vi "User Interface.vi"(10 "Test File Path":path=path "") -> ()   [LabVIEW 2020, in "Execution UI V2.lvclass"]
uses:
  Execution UI V2.lvclass
  <vilib>/Utility/miscctls.llb/LVNodeAndColumnTypeDef.ctl
  Application Framework/Process Classes/Process/Process.lvclass/Process.ctl
  Private/TypeDefs/Execution State.ctl
  Execution UI V2.lvclass/Execution UI V2.ctl
  Framework/Result Types/Case Result/Test Case Result.ctl
  Framework/Result Types/Method Result/Method Result.ctl
  Result/Status.ctl
  Framework/Result Types/Assertion Result/Assertion Result.ctl
  Framework/Result Types/Assertion Result/Public/TypeDefs/Assertion Type.ctl
  Framework/Result Types/Suite Results/Test Suite Result.ctl
  Result Model/Tree Item Filter.ctl
  Test Tree/Test Tree.lvclass
  Application Framework/Process Classes/Process/Public/Accessors/Read Process Name.vi
  C:/Git/astemes-lunit/source/Application Framework/Process Classes/Process/Process.lvclass
  <vilib>/Utility/error.llb/Error Cluster From Error Code.vi
  Framework/Result View/Result View.vi
  Application Framework/Process Classes/Error Handler/Private/SubVIs/Get Error Queue Name.vi
  <vilib>/Platform/browser.llb/Open URL in Default Browser (string).vi
  Framework/Result Types/Case Result/Test Case Result.lvlib
  Framework/Result Types/Method Result/Method Result.lvlib
  Framework/Result Types/Suite Results/Test Suite Result.lvlib
  Application Framework/Process Classes/Process/Process.lvclass
  Application Framework/Process Classes/Error Handler/Error Handler.lvclass
  Framework/Test Result View/Test Result View.lvclass
  Framework/Result Types/Assertion Result/Assertion Result.lvlib
  Result/Result.lvlib
  Result Table/Result Table V2.lvclass
  Result Model/Result Model.lvclass
panel:
  in  "Refresh":bool
  in  "Run Single Test":bool
  in  "Stop":bool
  in  "Run All Tests":bool
  in  "Eject":bool
  in  "Save":bool
  in  "Collapse":bool
  in  "Expand":bool
  out "Progress bar":dbl(slide) scale=0.0..100.0
  out "Results":i32(listbox)=-1
  in  "Test Results":string[](tree)
  in  "Filter fails":bool
  out "Description":string
  out "Status":string
  out "error out":errorcluster
  in  "error in (no error)":errorcluster
  # "1"
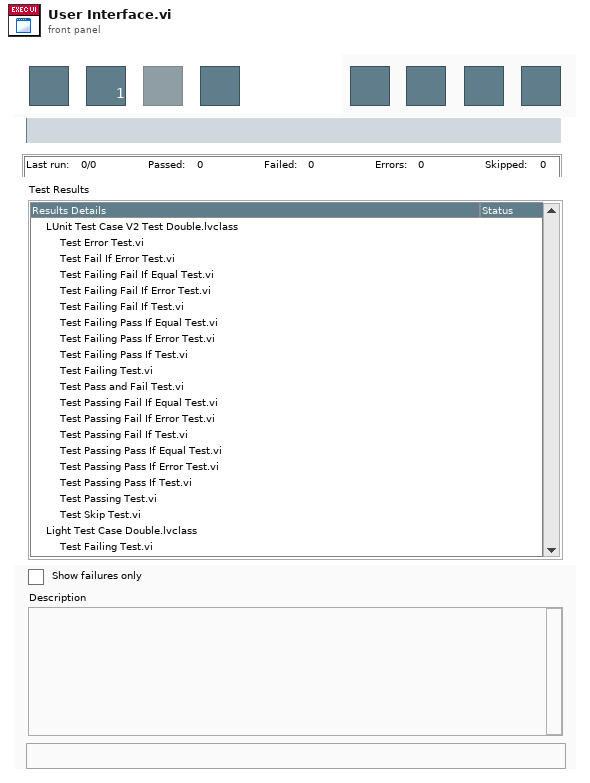
[diagram p1: front panel]
types:
  T1 = typedef "Execution UI V2.lvclass/Execution State.ctl" = enum16{"Idle", "Running"}
  T2 = typedef "Test Case Result.lvlib/Test Case Result.ctl" = map{string, T3}
  T3 = typedef "Method Result.lvlib/Method Result.ctl" = cluster{"Test Case":string, "Test Method Name":string, "Status":T4, "Assertion Results":T5[], "Execution time":dbl, "Result String":string}
  T4 = typedef "Result.lvlib/Status.ctl" = enum16{"", "Passed", "Failed", "Error", "Skipped", "Setup Error", "Broken", "Teardown Error"}
  T5 = typedef "Assertion Result.lvlib/Assertion Result.ctl" = cluster{"Status":T4, "Message":string, "Description":string, "Assertion Type":T6}
  T6 = typedef "Result.lvlib/Assertion Type.ctl" = enum16{"None", "Pass", "Fail", "Skip", "Pass if Equal", "Fail if Equal", "Pass if Error", "Fail if Error", "Pass if", "Fail if"}
  T7 = typedef "Test Suite Result.lvlib/Test Suite Result.ctl" = cluster{"Test Suite ID":string, "Name":string, "Hostname":string, "Status":T4, "Execution time":dbl, "Start Time":timestamp, "Case Results":T2[]}
  T8 = typedef "Result Model.lvclass/Tree Item Filter.ctl" = enum16{"All", "Only Fails"}
  T9 = typedef "LVNodeAndColumnTypeDef.ctl" = cluster{"Node":string, "Column":i32}
  T10 = enum8{"Enabled", "Disabled", "Disabled and Grayed Out"}
  T11 = typedef "Assertion Result.lvlib/Status.ctl" = enum16{"Pass", "Fail", "Error", "Skipped", "Setup Error", "Broken", "Teardown Error"}
  T12 = enum32{"Invalid", "Standard", "Closed", "Hidden", "Minimized", "Maximized"}
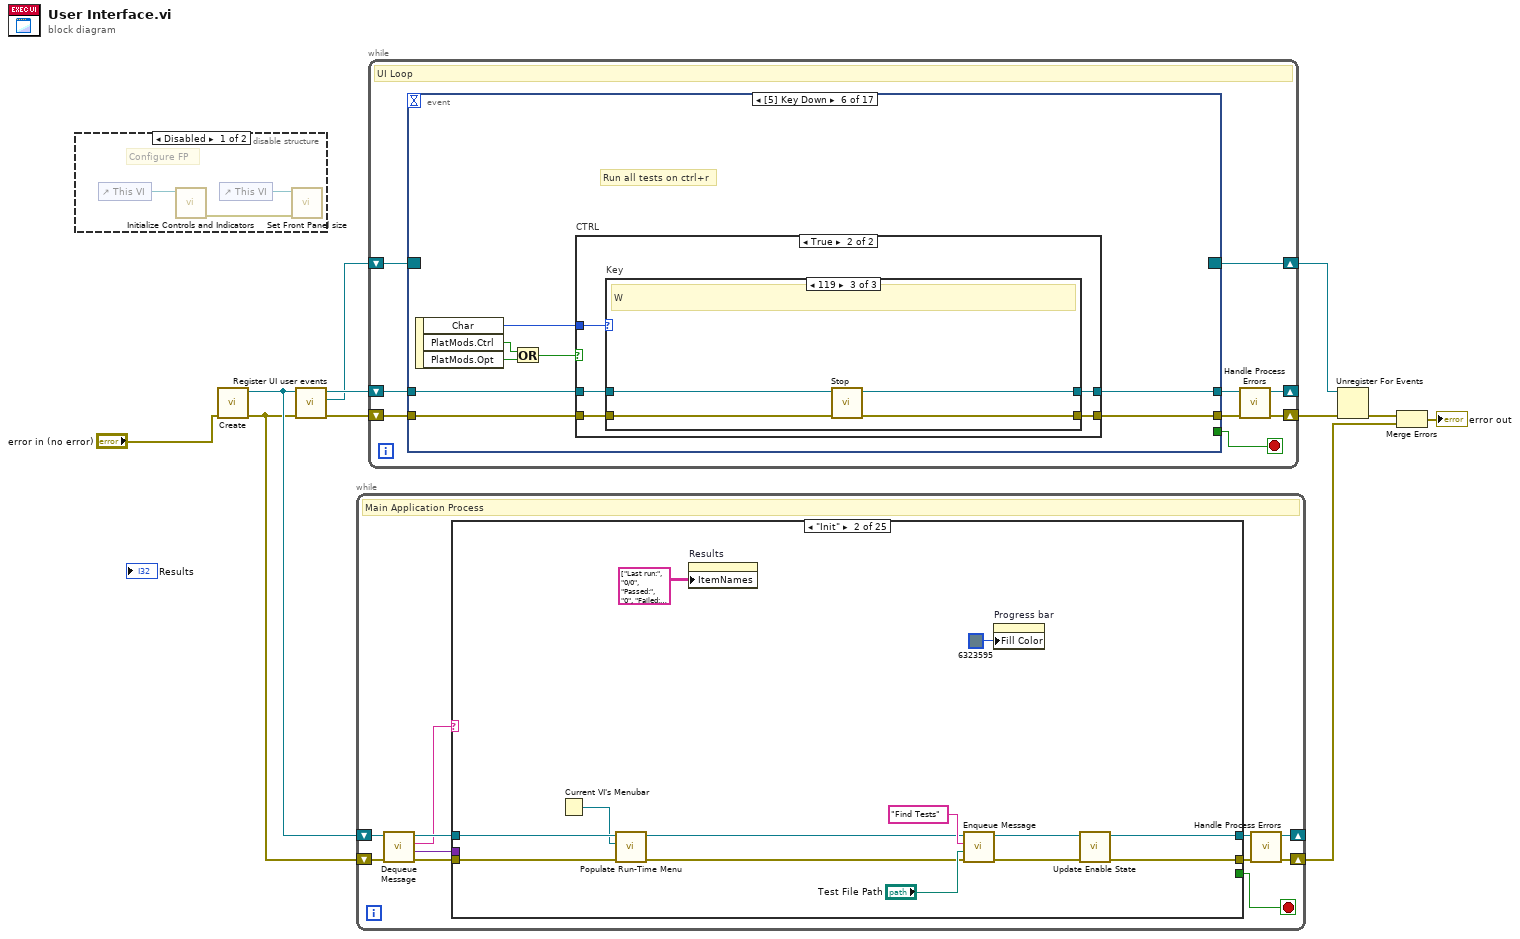
[diagram p0: block diagram]
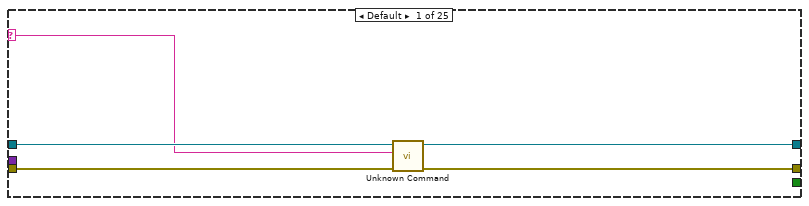
[diagram p2: hidden frame]
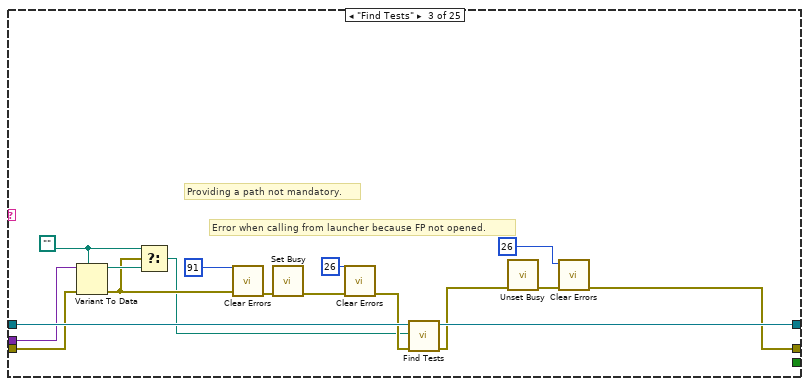
[diagram p3: hidden frame]
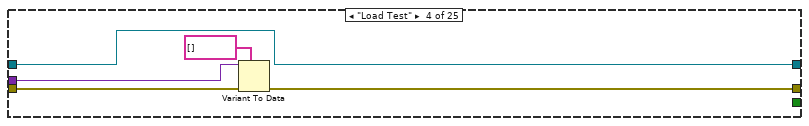
[diagram p4: hidden frame]
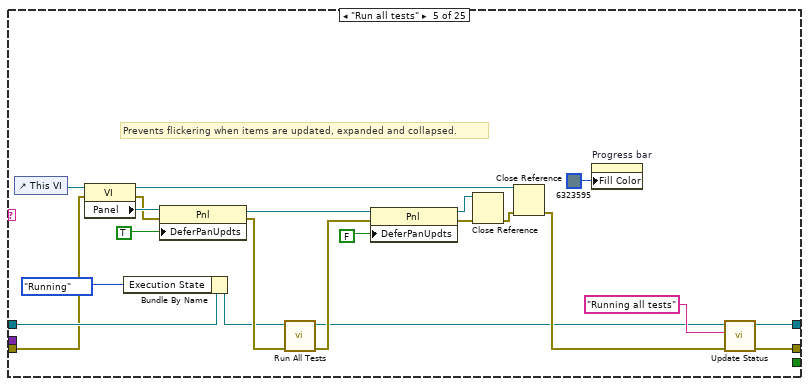
[diagram p5: hidden frame]
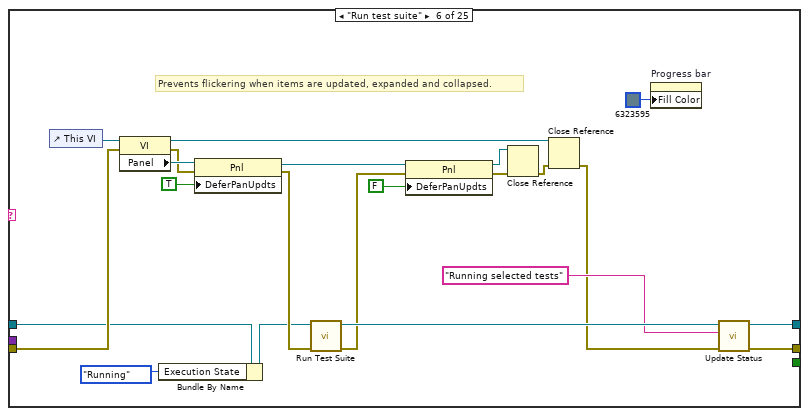
[diagram p6: hidden frame]
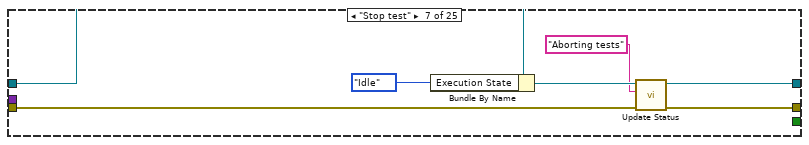
[diagram p7: hidden frame]
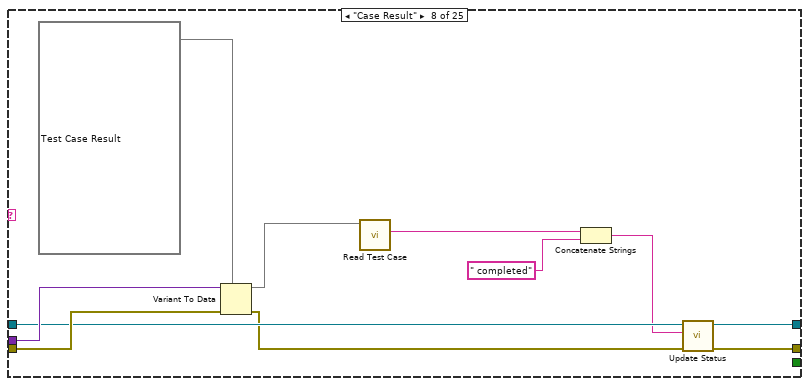
[diagram p8: hidden frame]
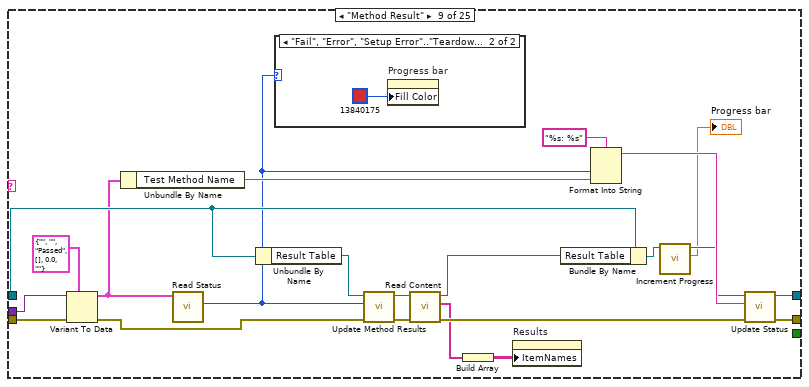
[diagram p9: hidden frame]
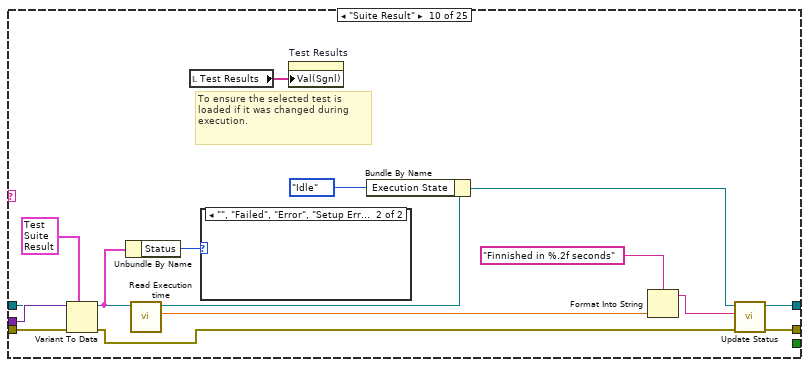
[diagram p11: hidden frame]
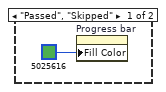
[diagram p12: hidden frame]
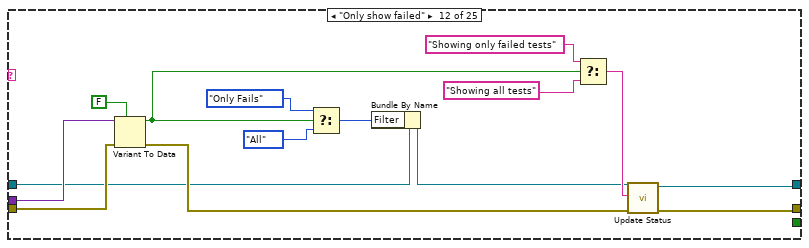
[diagram p14: hidden frame]
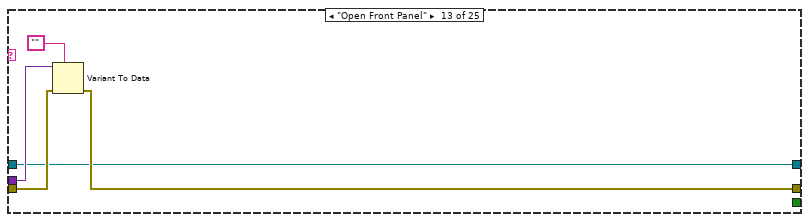
[diagram p15: hidden frame]
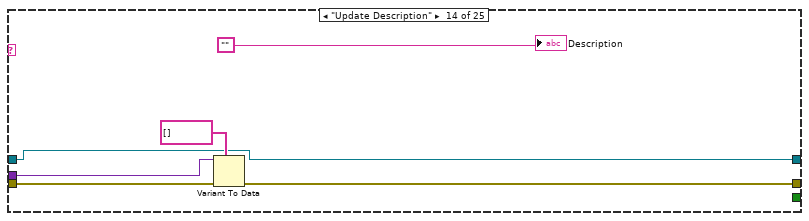
[diagram p16: hidden frame]
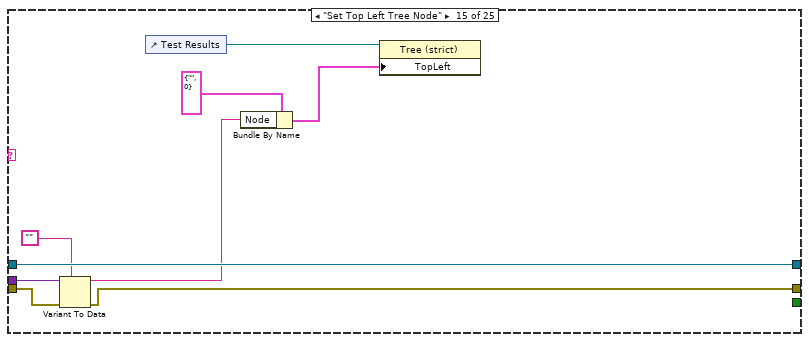
[diagram p17: hidden frame]
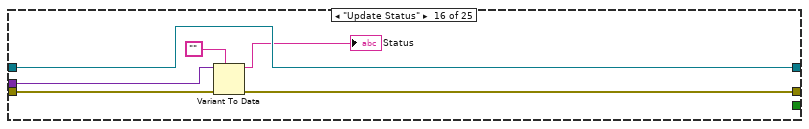
[diagram p18: hidden frame]
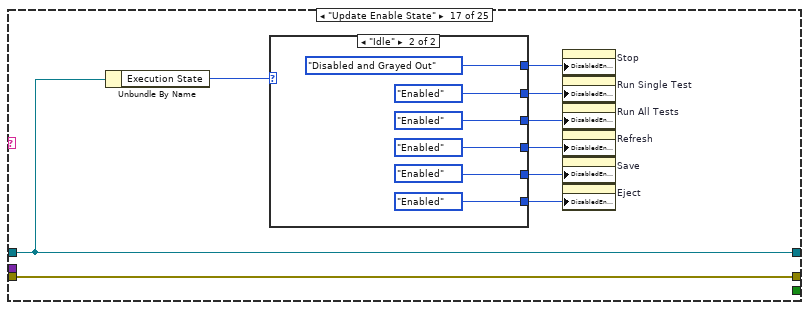
[diagram p19: hidden frame]
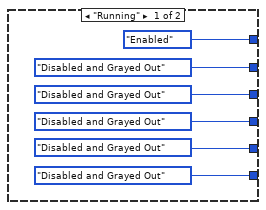
[diagram p20: hidden frame]
diagram:
  n1 = disable-structure shown="Disabled" {
    frame Disabled {
      # "Configure FP"
      n2 = control-ref of="This VI"() -> (w13:refnum<vi>)
      n3 = call "Initialize Controls and Indicators.vi"("VI in"=w13) -> ("error out"=w12:errorcluster)  [unwired: 10 in]
      n4 = control-ref of="This VI"() -> (w14:refnum<vi>)
      n5 = call "Set Front Panel size.vi"("error in (no error)"=w12, "VI in"=w14) -> ()  [unwired: 9 in, 1 out]
    }
    frame Enabled {
    }
  }
  n6 = call "Create.vi"("error in (no error)"="error in (no error)") -> ("error out"=w5:errorcluster, "Execution UI Out"=w6:refnum<class "Execution UI V2.lvclass">)  [unwired: 9 in]
  n7 = call "Register UI user events.vi"("error in (no error)"=w5, "Execution UI In"=w6) -> ("error out"=w10:errorcluster, "Event Registration Refnum"=w8:refnum<event-registration>, "Execution UI Out"=w11:refnum<class "Execution UI V2.lvclass">)  [unwired: 7 in]
  n8 = while {
    shift-right: [w16] -> w7
    shift-left: w5 -> [w24]
    shift-right: [w17] -> _
    shift-left: w6 -> [w25]
    stop <- w20 stop-if-true
    # "Main Application Process"
    n9 = call "Dequeue Message.vi"("error in (no error)"=w24, "Process In"=w25) -> ("error out"=w22:errorcluster, "Message Data"=w18:variant, "Message"=w19:string, "Process Out"=w23:refnum<class "Execution UI V2.lvclass">)  [unwired: 6 in]
    n10 = case shown="\"Init\"" w19 {
      selector: w19 -> [w26 _ _ _ _ _ _ _ _ _ _ _ _ _ _ _ _ _ w246 _ _ _ _ _ _]
      tunnel: w23 -> [w27 w35 w60 w65 w87 w89 w115 w124 w142 w158 w168 w174 w184 w190 w202 w206 w217 w244 w252 w259 w267 w275 w283 w289 w298]
      tunnel: [w28 w40 w57 w65 w86 w108 w110 w123 w146 w163 w168 w179 w184 w190 w202 w206 w217 w244 w252 w257 w265 w273 w281 w286 w302] -> w21
      tunnel: w22 -> [w29 w36 w53 w61 w79 w90 w114 w127 w149 w165 w167 w183 w188 w194 w203 w209 w218 w242 w251 w253 w264 w272 w280 w290 w292]
      tunnel: [w30 w39 w45 w62 w85 w107 w113 w122 w145 w162 w167 w178 w185 w191 w199 w205 w218 w243 w250 w258 w266 w274 w282 w285 w301] -> w15
      tunnel: [_ _ _ _ _ _ _ _ _ _ _ _ _ _ _ _ _ _ _ _ _ _ _ _ TRUE] -> w20
      tunnel: w18 -> [_ _ w56 w64 _ _ _ w126 w148 w164 _ w182 w187 w193 w201 w208 _ _ w249 _ _ _ _ _ _]
      frame Default {
        n11 = call "Unknown Command.vi"("error in (no error)"=w29, "String"=w26, "Process In"=w27) -> ("error out"=w30:errorcluster, "Process Out"=w28:refnum<class "Execution UI V2.lvclass">)  [unwired: 7 in]
      }
      frame "Init" {
        n12 = Current VI's Menubar() -> (w32:refnum<k9>)
        n13 = call "Populate Run-Time Menu.vi"("error in (no error)"=w36, "Menu in"=w32, "Execution UI"=w35) -> ("error out"=w34:errorcluster, "Execution UI"=w33:refnum<class "Execution UI V2.lvclass">)  [unwired: 7 in]
        n14 = property on="Results" class="MCListbox (strict)"("ItemNames"=string[][] [["Last run:", "0/0", "Passed:", "0", "Failed:", "0", "Errors:", "0", "Skipped:", "0"]] ("Result Texts")) -> ()  [unwired: 2 in, 2 out]
        n15 = call "Enqueue Message.vi"("error in (no error)"=w34, "Message Data"="Test File Path", "Message"="Find Tests", "Process In"=w33) -> ("error out"=w41:errorcluster, "Process Out"=w42:refnum<class "Execution UI V2.lvclass">)  [unwired: 6 in]
        n16 = property on="Progress bar" class="Slide (strict)"("Fill Color"=u32 6323595) -> ()  [unwired: 2 in, 2 out]
        n17 = call "Update Enable State.vi"("error in (no error)"=w41, "Execution UI In"=w42) -> ("error out"=w39:errorcluster, "Execution UI Out"=w40:refnum<class "Execution UI V2.lvclass">)  [unwired: 8 in]
      }
      frame "Find Tests" {
        w55 = path "" ("Not A Path Constant")
        # "Error when calling from launcher because FP not opened."
        # "Providing a path not mandatory."
        n18 = Variant To Data(error in=w53, type=w55, Variant=w56) -> (data=w54:path, error out=w50:errorcluster)
        n19 = Select(t=w55, s=w50, f=w54) -> (s? t:f=w44:path)
        n20 = call <vilib>:"Clear Errors.vi"("error in (no error)"=w50, "specific error code to clear (0: all)"=91) -> ("error out"=w52:errorcluster)  [unwired: 4 in, 1 out]
        n21 = call <vilib>:"Set Busy.vi"("error in (no error)"=w52) -> ("error out"=w59:errorcluster)  [unwired: 9 in, 1 out]
        n22 = call <vilib>:"Clear Errors.vi"("error in (no error)"=w59, "specific error code to clear (0: all)"=26) -> ("error out"=w49:errorcluster)  [unwired: 4 in, 1 out]
        n23 = call "Find Tests.vi"("error in (no error)"=w49, "Project or Class Path"=w44, "Execution UI In"=w60) -> ("error out"=w46:errorcluster, "Execution UI Out"=w57:refnum<class "Execution UI V2.lvclass">)  [unwired: 7 in]
        n24 = call <vilib>:"Unset Busy.vi"("error in (no error)"=w46) -> ("error out"=w58:errorcluster)  [unwired: 10 in]
        n25 = call <vilib>:"Clear Errors.vi"("error in (no error)"=w58, "specific error code to clear (0: all)"=26) -> ("error out"=w45:errorcluster)  [unwired: 4 in, 1 out]
      }
      frame "Load Test" {
        n26 = Variant To Data(error in=w61, type=string[] [], Variant=w64) -> (error out=w62:errorcluster)  [unwired: 1 out]
      }
      frame "Run all tests" {
        # "Prevents flickering when items are updated, expanded and collapsed."
        n27 = control-ref of="This VI"() -> (w83:refnum<vi>)
        n28 = property on="Property Node" class="VI"(reference=w83, error in=w79) -> (reference out=w73:refnum<vi>, error out=w81:errorcluster, "Panel"=w82:refnum<vi>)
        n29 = Bundle By Name(cluster=w87, "Execution State"=Execution_State."Running") -> (w69:refnum<class "Execution UI V2.lvclass">)
        n30 = property on="Property Node" class="Pnl"(reference=w82, error in=w81, "DeferPanUpdts"=TRUE ("Defer Panel Updates")) -> (reference out=w74:refnum<vi>, error out=w80:errorcluster)
        n31 = call "Run All Tests.vi"("error in (no error)"=w80, "Execution UI In"=w69) -> ("error out"=w72:errorcluster, "Execution UI Out"=w67:refnum<class "Execution UI V2.lvclass">)  [unwired: 8 in]
        n32 = property on="Property Node" class="Pnl"(reference=w74, error in=w72, "DeferPanUpdts"=FALSE ("Defer Panel Updates")) -> (reference out=w75:refnum<vi>, error out=w77:errorcluster)
        n33 = Close Reference(reference=w75, error in (no error)=w77) -> (error out=w76:errorcluster)
        n34 = Close Reference(reference=w73, error in (no error)=w76) -> (error out=w71:errorcluster)
        n35 = property on="Progress bar" class="Slide (strict)"("Fill Color"=u32 6323595) -> ()  [unwired: 2 in, 2 out]
        n36 = call "Update Status.vi"("error in (no error)"=w71, "Status"="Running all tests", "Execution UI In"=w67) -> ("error out"=w85:errorcluster, "Execution UI Out"=w86:refnum<class "Execution UI V2.lvclass">)  [unwired: 7 in]
      }
      frame "Run test suite" {
        # "Prevents flickering when items are updated, expanded and collapsed."
        n37 = control-ref of="This VI"() -> (w105:refnum<vi>)
        n38 = property on="Property Node" class="VI"(reference=w105, error in=w90) -> (reference out=w97:refnum<vi>, error out=w103:errorcluster, "Panel"=w104:refnum<vi>)
        n39 = Bundle By Name(cluster=w89, "Execution State"=Execution_State."Running") -> (w92:refnum<class "Execution UI V2.lvclass">)
        n40 = property on="Property Node" class="Pnl"(reference=w104, error in=w103, "DeferPanUpdts"=TRUE ("Defer Panel Updates")) -> (reference out=w98:refnum<vi>, error out=w95:errorcluster)
        n41 = call "Run Test Suite.vi"("error in (no error)"=w95, "Execution UI In"=w92) -> ("error out"=w94:errorcluster, "Execution UI Out"=w109:refnum<class "Execution UI V2.lvclass">)  [unwired: 8 in]
        n42 = property on="Property Node" class="Pnl"(reference=w98, error in=w94, "DeferPanUpdts"=FALSE ("Defer Panel Updates")) -> (reference out=w99:refnum<vi>, error out=w101:errorcluster)
        n43 = Close Reference(reference=w99, error in (no error)=w101) -> (error out=w100:errorcluster)
        n44 = Close Reference(reference=w97, error in (no error)=w100) -> (error out=w93:errorcluster)
        n45 = property on="Progress bar" class="Slide (strict)"("Fill Color"=u32 6323595) -> ()  [unwired: 2 in, 2 out]
        n46 = call "Update Status.vi"("error in (no error)"=w93, "Status"="Running selected tests", "Execution UI In"=w109) -> ("error out"=w107:errorcluster, "Execution UI Out"=w108:refnum<class "Execution UI V2.lvclass">)  [unwired: 7 in]
      }
      frame "Stop test" {
        n47 = Bundle By Name(cluster=w115, "Execution State"=Execution_State."Idle") -> (w116:refnum<class "Execution UI V2.lvclass">)
        n48 = call "Update Status.vi"("error in (no error)"=w114, "Status"="Aborting tests", "Execution UI In"=w116) -> ("error out"=w113:errorcluster, "Execution UI Out"=w110:refnum<class "Execution UI V2.lvclass">)  [unwired: 7 in]
      }
      frame "Case Result" {
        n49 = Variant To Data(error in=w127, type=T2 {} ("Case Result"), Variant=w126) -> (data=w120:T2, error out=w117:errorcluster)
        n50 = call "Read Test Case.vi"("Test Case Result In"=w120) -> ("Test Case"=w118:string)  [unwired: 9 in, 1 out]
        n51 = Concatenate Strings(w118, " completed" ("Status")) -> (w119:string)
        n52 = call "Update Status.vi"("error in (no error)"=w117, "Status"=w119, "Execution UI In"=w124) -> ("error out"=w122:errorcluster, "Execution UI Out"=w123:refnum<class "Execution UI V2.lvclass">)  [unwired: 7 in]
      }
      frame "Method Result" {
        n53 = Variant To Data(error in=w149, type=T3 {"Test Case"="", "Test Method Name"="", "Status"=enum."Passed", "Assertion Results"=[], "Execution time"=0.0, "Result String"=""} ("Test Method Result.lvclass"), Variant=w148) -> (data=w134:T3, error out=w137:errorcluster)
        n54 = Unbundle By Name(w134) -> ("Test Method Name"=w135:string)
        n55 = call "Read Status.vi"("Method Result In"=w134) -> ("Status"=w130:T11)  [unwired: 8 in, 2 out]
        n56 = Unbundle By Name(w142) -> ("Result Table"=w129:refnum<class "Result Table V2.lvclass">)
        n57 = case shown="\"Fail\", \"Error\", \"Setup Error\"..\"Teardown Error\"" w130 {
          frame "Pass", "Skipped" {
          }
          frame "Fail", "Error", "Setup Error".."Teardown Error" {
            n58 = property on="Progress bar" class="Slide (strict)"("Fill Color"=u32 13840175) -> ()  [unwired: 2 in, 2 out]
          }
        }
        n59 = call "Update Method Results.vi"("error in (no error)"=w137, "Method Result"=w130, "Result Table in"=w129) -> ("error out"=w138:errorcluster, "Result Table out"=w132:refnum<class "Result Table V2.lvclass">)  [unwired: 7 in]
        n60 = call "Read Content.vi"("error in (no error)"=w138, "Result Table in"=w132) -> ("error out"=w133:errorcluster, "Result Texts"=w131:string[], "Result Table out"=w128:refnum<class "Result Table V2.lvclass">)  [unwired: 7 in]
        n61 = Build Array(w131) -> (w136:string[][])
        n62 = property on="Results" class="MCListbox (strict)"("ItemNames"=w136) -> ()  [unwired: 2 in, 2 out]
        n63 = Bundle By Name(cluster=w142, "Result Table"=w128) -> (w141:refnum<class "Execution UI V2.lvclass">)
        n64 = Format Into String(format string="%s: %s", w130, w135) -> (resulting string=w143:string)  [unwired: 2 in, 1 out]
        n65 = call "Increment Progress.vi"("Execution UI In"=w141) -> ("Progress (%)"=→"Progress bar":dbl, "Execution UI Out"=w140:refnum<class "Execution UI V2.lvclass">)  [unwired: 9 in]
        n66 = call "Update Status.vi"("error in (no error)"=w133, "Status"=w143, "Execution UI In"=w140) -> ("error out"=w145:errorcluster, "Execution UI Out"=w146:refnum<class "Execution UI V2.lvclass">)  [unwired: 7 in]
      }
      frame "Suite Result" {
        # "To ensure the selected test is loaded if it was changed during execution."
        n67 = Variant To Data(error in=w165, type=T7 {"Test Suite ID"="", "Name"="", "Hostname"="", "Status"=enum."Passed", "Execution time"=0.0, "Start Time"=timestamp(0 s since 1904-01-01), "Case Results"=[]} ("Cluster of class private data"), Variant=w164) -> (data=w152:T7, error out=w154:errorcluster)
        n68 = Unbundle By Name(w152) -> ("Status"=w151:T4)
        n69 = call "Read Execution time.vi"("Test Suite Result In"=w152) -> ("Execution time"=w160:dbl)  [unwired: 8 in, 2 out]
        n70 = local read "Test Results"() -> (w155:string[])
        n71 = case shown="\"\", \"Failed\", \"Error\", \"Setup Error\"..\"Teardown Error\"" w151 {
          frame "Passed", "Skipped" {
            n72 = property on="Progress bar" class="Slide (strict)"("Fill Color"=u32 5025616) -> ()  [unwired: 2 in, 2 out]
          }
          frame "", "Failed", "Error", "Setup Error".."Teardown Error" {
          }
        }
        n73 = property on="Test Results" class="Tree (strict)"("Val(Sgnl)"=w155) -> ()  [unwired: 2 in, 2 out]
        n74 = Bundle By Name(cluster=w158, "Execution State"=Execution_State."Idle") -> (w157:refnum<class "Execution UI V2.lvclass">)
        n75 = Format Into String(format string="Finnished in %.2f seconds", w160) -> (resulting string=w159:string)  [unwired: 2 in, 1 out]
        n76 = call "Update Status.vi"("error in (no error)"=w154, "Status"=w159, "Execution UI In"=w157) -> ("error out"=w162:errorcluster, "Execution UI Out"=w163:refnum<class "Execution UI V2.lvclass">)  [unwired: 7 in]
      }
      frame "Save results" {
        # "#TODO"
      }
      frame "Only show failed" {
        n77 = Variant To Data(error in=w183, type=FALSE, Variant=w182) -> (data=w172:bool, error out=w180:errorcluster)
        n78 = Select(t=Tree_Item_Filter."Only Fails" ("Filter"), s=w172, f=Tree_Item_Filter."All" ("Filter")) -> (s? t:f=w169:T8)
        n79 = Bundle By Name(cluster=w174, "Filter"=w169) -> (w173:refnum<class "Execution UI V2.lvclass">)
        n80 = Select(t="Showing only failed tests" ("Status"), s=w172, f="Showing all tests" ("Status")) -> (s? t:f=w177:string)
        n81 = call "Update Status.vi"("error in (no error)"=w180, "Status"=w177, "Execution UI In"=w173) -> ("error out"=w178:errorcluster, "Execution UI Out"=w179:refnum<class "Execution UI V2.lvclass">)  [unwired: 7 in]
      }
      frame "Open Front Panel" {
        n82 = Variant To Data(error in=w188, type="" ("Empty String Constant"), Variant=w187) -> (error out=w185:errorcluster)  [unwired: 1 out]
      }
      frame "Update Description" {
        n83 = Variant To Data(error in=w194, type=string[] [], Variant=w193) -> (error out=w191:errorcluster)  [unwired: 1 out]
        "Description" <- "" ("Empty String Constant")
      }
      frame "Set Top Left Tree Node" {
        n84 = Variant To Data(error in=w203, type="", Variant=w201) -> (data=w195:string, error out=w199:errorcluster)
        n85 = control-ref of="Test Results"() -> (w198:refnum<vi>)
        n86 = Bundle By Name(cluster=T9 {"Node"="", "Column"=0} ("Top Left Visible Cell"), "Node"=w195) -> (w196:T9)
        n87 = property on="Property Node" class="Tree (strict)"(reference=w198, "TopLeft"=w196) -> ()  [unwired: 1 in, 2 out]
      }
      frame "Update Status" {
        n88 = Variant To Data(error in=w209, type="" ("Empty String Constant"), Variant=w208) -> (data=→"Status":string, error out=w205:errorcluster)
      }
      frame "Update Enable State" {
        n89 = Unbundle By Name(w217) -> ("Execution State"=w216:T1)
        n90 = case shown="\"Idle\"" w216 {
          tunnel: [T10."Enabled" ("Disabled") T10."Disabled and Grayed Out" ("Disabled")] -> w215
          tunnel: [T10."Disabled and Grayed Out" ("Disabled") T10."Enabled" ("Disabled")] -> w214
          tunnel: [T10."Disabled and Grayed Out" ("Disabled") T10."Enabled" ("Disabled")] -> w213
          tunnel: [T10."Disabled and Grayed Out" ("Disabled") T10."Enabled" ("Disabled")] -> w212
          tunnel: [T10."Disabled and Grayed Out" ("Disabled") T10."Enabled" ("Disabled")] -> w211
          tunnel: [T10."Disabled and Grayed Out" ("Disabled") T10."Enabled" ("Disabled")] -> w210
          frame "Running" {
          }
          frame "Idle" {
          }
        }
        n91 = property on="Stop" class="Bool"("DisabledEnum"=w215) -> ()  [unwired: 2 in, 2 out]
        n92 = property on="Run Single Test" class="Bool"("DisabledEnum"=w214) -> ()  [unwired: 2 in, 2 out]
        n93 = property on="Run All Tests" class="Bool"("DisabledEnum"=w213) -> ()  [unwired: 2 in, 2 out]
        n94 = property on="Refresh" class="Bool"("DisabledEnum"=w212) -> ()  [unwired: 2 in, 2 out]
        n95 = property on="Save" class="Bool"("DisabledEnum"=w211) -> ()  [unwired: 2 in, 2 out]
        n96 = property on="Eject" class="Bool"("DisabledEnum"=w210) -> ()  [unwired: 2 in, 2 out]
      }
      frame "Launch Results View" {
        # "#TODO"
        n97 = vi-ref "Test Result View.lvclass:Result View.vi"() -> (w239:refnum<vi>)
        n98 = property class="VI"(reference=w239, error in=w242) -> (error out=w234:errorcluster, "Path"=w238:path)  [unwired: 1 out]
        n99 = Open VI Reference(type specifier VI Refnum (for type only)=refnum<vi> refnum, vi path=w238, options=128, error in (no error)=w234) -> (vi reference=w235:refnum<vi>, error out=w237:errorcluster)  [unwired: 2 in]
        n100 = call-by-ref "Start Asynchronous Call"(reference=w235, error in=w237, "TestCase map"=map{string, map{string, path}} {}, "Test Tree"=refnum<class "Test Tree.lvclass"> refnum) -> (reference out=w240:refnum<vi>, error out=w241:errorcluster)  [unwired: 10 in]
        n101 = Close Reference(reference=w240, error in (no error)=w241) -> (error out=w243:errorcluster)
      }
      frame "Ignore Inherited Tests" {
        # "#TODO \nSave selection to config"
        n102 = Variant To Data(error in=w251, type=FALSE, Variant=w249) -> (data=w245:bool, error out=w250:errorcluster)
        n103 = Current VI's Menubar() -> (w247:refnum<k9>)
        n104 = Set Menu Item Info(7:w246, 9:w245, 11:w247) -> ()  [unwired: 4 in, 2 out]
      }
      frame "Enable Execution Profiler" {
        # "#TODO"
        n105 = Current VI's Menubar() -> (w256:refnum<k9>)
        n106 = Set Menu Item Info(6:TRUE ("checked"), 7:"Execution Profiler...", 11:w256) -> ()  [unwired: 4 in, 2 out]
        n107 = call "Update Status.vi"("error in (no error)"=w253, "Status"="Run a test to generate an execution analysis.", "Execution UI In"=w259) -> ("error out"=w258:errorcluster, "Execution UI Out"=w257:refnum<class "Execution UI V2.lvclass">)  [unwired: 7 in]
      }
      frame "Enable Coverage Analyzer" {
        # "#TODO"
        n108 = Current VI's Menubar() -> (w263:refnum<k9>)
        n109 = Set Menu Item Info(6:TRUE ("checked"), 7:"Coverage Analyzer...", 11:w263) -> ()  [unwired: 4 in, 2 out]
        n110 = call "Update Status.vi"("error in (no error)"=w264, "Status"="Run a test to generate coverage analysis...", "Execution UI In"=w267) -> ("error out"=w266:errorcluster, "Execution UI Out"=w265:refnum<class "Execution UI V2.lvclass">)  [unwired: 7 in]
      }
      frame "Disable Execution Profiler" {
        # "#TODO"
        n111 = Current VI's Menubar() -> (w271:refnum<k9>)
        n112 = call "Update Status.vi"("error in (no error)"=w272, "Status"="Execution profiler disabled.", "Execution UI In"=w275) -> ("error out"=w274:errorcluster, "Execution UI Out"=w273:refnum<class "Execution UI V2.lvclass">)  [unwired: 7 in]
        n113 = Set Menu Item Info(6:FALSE ("checked"), 7:"Execution Profiler...", 11:w271) -> ()  [unwired: 4 in, 2 out]
      }
      frame "Disable Coverage Analyzer" {
        # "#TODO"
        n114 = Current VI's Menubar() -> (w279:refnum<k9>)
        n115 = call "Update Status.vi"("error in (no error)"=w280, "Status"="Coverage analyzer disabled.", "Execution UI In"=w283) -> ("error out"=w282:errorcluster, "Execution UI Out"=w281:refnum<class "Execution UI V2.lvclass">)  [unwired: 7 in]
        n116 = Set Menu Item Info(6:FALSE ("checked"), 7:"Coverage Analyzer...", 11:w279) -> ()  [unwired: 4 in, 2 out]
      }
      frame "Stop" {
        n117 = call "Enqueue Message.vi"("error in (no error)"=w290, "Message"="Exit", "Process In"=w289) -> ("error out"=w291:errorcluster, "Process Out"=w287:refnum<class "Execution UI V2.lvclass">)  [unwired: 7 in]
        n118 = call "Stop Processes.vi"("error in (no error)"=w291, "Execution UI In"=w287) -> ("error out"=w285:errorcluster, "Execution UI Out"=w286:refnum<class "Execution UI V2.lvclass">)  [unwired: 8 in]
      }
      frame "Exit" {
        n119 = control-ref of="This VI"() -> (w296:refnum<vi>)
        n120 = invoke on="Invoke Node" class="VI" method="FP.Close"(reference=w296, error in=w292) -> (reference out=w294:refnum<vi>, error out=w295:errorcluster)  [unwired: 1 in, 1 out]
        n121 = Close Reference(reference=w294, error in (no error)=w295) -> (error out=w293:errorcluster)
        n122 = call "Finish.vi"("error in (no error)"=w293, "Process In"=w298) -> ("error out"=w297:errorcluster, "Process Out"=w299:refnum<class "Execution UI V2.lvclass">)  [unwired: 8 in]
        n123 = call-dynamic "Clear.vi"("error in (no error)"=w297, "Execution UI In"=w299) -> ("error out"=w301:errorcluster, "Execution UI Out"=w302:refnum<class "Execution UI V2.lvclass">)  [unwired: 8 in]
      }
    }
    n124 = call "Handle Process Errors.vi"("error in (no error)"=w15, "Process In"=w21) -> ("error out"=w16:errorcluster, "Process Out"=w17:refnum<class "Execution UI V2.lvclass">)  [unwired: 8 in]
  }
  n125 = while {
    shift-right: [w303] -> w4
    shift-left: w10 -> [w310]
    shift-right: [w305] -> _
    shift-left: w11 -> [w311]
    shift-right: [w307] -> w9
    shift-left: w8 -> [w306]
    stop <- w308 stop-if-true
    # "UI Loop"
    n126 = event shown="[5] Key Down" {
      selector: w306 -> [_ _ _ _ _ _ _ _ _ _ _ _ _ _ _ _ _]
      dyn-events: [_ _ _ _ _ _ _ _ _ _ _ _ _ _ _ _ _] -> w307
      timeout: _ -> [_ _ _ _ _ _ _ _ _ _ _ _ _ _ _ _ _]
      tunnel: w311 -> [w317 w320 w327 w331 w337 w347 w372 w379 w389 w394 w398 w408 w419 w427 w462 w570 w576]
      tunnel: w310 -> [w318 w321 w325 w329 w339 w348 w374 w382 w388 w392 w396 w407 w409 w420 w461 w571 w573]
      tunnel: [w318 w321 w324 w330 w336 w346 w371 w378 w386 w391 w397 w406 w410 w425 w460 w571 w574] -> w304
      tunnel: [w317 w320 w326 w332 w334 w345 w369 w376 w387 w393 w399 w405 w419 w424 w459 w570 w575] -> w309
      tunnel: [_ _ _ _ _ _ _ _ _ _ _ _ _ _ _ TRUE _] -> w308
      event "Collapse": Value Change {
        n127 = event-data() -> ()  [unwired: 1 in, 6 out]
        n128 = property on="Test Results" class="Tree (strict)"() -> ("All Tags"=w315:string[])  [unwired: 2 in, 2 out]
        n129 = invoke on="Test Results" class="Tree (strict)" method="Open/Close.Open/Close All"("Open"=FALSE ("Open?")) -> ()  [unwired: 3 in, 4 out]
        n130 = Index Array(array=w315) -> (element=w312:string)  [unwired: 1 in]
        n131 = Bundle By Name(cluster=T9 {"Node"="", "Column"=0} ("Top Left Visible Cell"), "Node"=w312) -> (w313:T9)
        n132 = property on="Test Results" class="Tree (strict)"("TopLeft"=w313) -> ()  [unwired: 2 in, 2 out]
      }
      event "Expand": Value Change {
        n133 = event-data() -> ()  [unwired: 1 in, 6 out]
        n134 = invoke on="Test Results" class="Tree (strict)" method="Open/Close.Open/Close All"("Open"=TRUE ("Open?")) -> ()  [unwired: 3 in, 4 out]
      }
      event "Filter fails": Value Change {
        n135 = event-data() -> ()  [unwired: 1 in, 1 out]
        n136 = call "Enqueue Message.vi"("error in (no error)"=w325, "Message Data"="Filter fails", "Message"="Only show failed", "Process In"=w327) -> ("error out"=w324:errorcluster, "Process Out"=w326:refnum<class "Execution UI V2.lvclass">)  [unwired: 6 in]
      }
      event "Refresh": Value Change {
        # "#TODO"
        n137 = event-data() -> ()  [unwired: 1 in, 1 out]
        n138 = call "Update Status.vi"("error in (no error)"=w329, "Status"="Recreating test case index.. ", "Execution UI In"=w331) -> ("error out"=w330:errorcluster, "Execution UI Out"=w332:refnum<class "Execution UI V2.lvclass">)  [unwired: 7 in]
        n139 = One Button Dialog(message="To do") -> ()  [unwired: 1 in, 1 out]
      }
      event "Run All Tests": Value Change {
        w338 = "Run all tests"  # Message
        # "#TODO"
        n140 = event-data() -> ()  [unwired: 1 in, 1 out]
        n141 = call "Enqueue Message.vi"("error in (no error)"=w339, "Message"=w338, "Process In"=w337) -> ("error out"=w340:errorcluster, "Process Out"=w335:refnum<class "Execution UI V2.lvclass">)  [unwired: 7 in]
        n142 = call "Update Enable State.vi"("error in (no error)"=w340, "Execution UI In"=w335) -> ("error out"=w336:errorcluster, "Execution UI Out"=w334:refnum<class "Execution UI V2.lvclass">)  [unwired: 8 in]
      }
      event Key Down {
        # "Run all tests on ctrl+r"
        n143 = event-data() -> ("Char"=w341:i16, "PlatMods.Ctrl"=w344:bool, "PlatMods.Opt"=w343:bool)  [unwired: 1 in]
        n144 = Or(x=w344, y=w343) -> (x .or. y?=w342:bool)
        n145 = case "CTRL" shown="True" w342 {
          tunnel: w348 -> [w349 w355]
          tunnel: w347 -> [w350 w354]
          tunnel: [w349 w353] -> w346
          tunnel: [w350 w352] -> w345
          tunnel: w341 -> [_ w351]
          frame False {
          }
          frame True {
            n146 = case "Key" shown="119" w351 {
              tunnel: w355 -> [w356 w363 w367]
              tunnel: w354 -> [w357 w361 w368]
              tunnel: [w356 w360 w365] -> w353
              tunnel: [w357 w358 w366] -> w352
              frame Default {
              }
              frame 114 {
                w362 = "Run all tests"  # Message
                # "R"
                n147 = call "Enqueue Message.vi"("error in (no error)"=w363, "Message"=w362, "Process In"=w361) -> ("error out"=w364:errorcluster, "Process Out"=w359:refnum<class "Execution UI V2.lvclass">)  [unwired: 7 in]
                n148 = call "Update Enable State.vi"("error in (no error)"=w364, "Execution UI In"=w359) -> ("error out"=w360:errorcluster, "Execution UI Out"=w358:refnum<class "Execution UI V2.lvclass">)  [unwired: 8 in]
              }
              frame 119 {
                # "W"
                n149 = call-dynamic "Stop.vi"("error in (no error)"=w367, "Execution UI In"=w368) -> ("error out"=w365:errorcluster, "Execution UI Out"=w366:refnum<class "Execution UI V2.lvclass">)  [unwired: 7 in, 1 out]
              }
            }
          }
        }
      }
      event "Run Single Test": Value Change {
        w373 = "Run test suite"  # Message
        # "#TODO"
        n150 = event-data() -> ()  [unwired: 1 in, 1 out]
        n151 = call "Enqueue Message.vi"("error in (no error)"=w374, "Message"=w373, "Process In"=w372) -> ("error out"=w375:errorcluster, "Process Out"=w370:refnum<class "Execution UI V2.lvclass">)  [unwired: 7 in]
        n152 = call "Update Enable State.vi"("error in (no error)"=w375, "Execution UI In"=w370) -> ("error out"=w371:errorcluster, "Execution UI Out"=w369:refnum<class "Execution UI V2.lvclass">)  [unwired: 8 in]
      }
      event "Stop": Value Change {
        n153 = event-data() -> ()  [unwired: 1 in, 2 out]
        n154 = call "Enqueue Message.vi"("error in (no error)"=w382, "Message"="Stop test", "Process In"=w379) -> ("error out"=w381:errorcluster, "Process Out"=w377:refnum<class "Execution UI V2.lvclass">)  [unwired: 7 in]
        n155 = call "Update Enable State.vi"("error in (no error)"=w381, "Execution UI In"=w377) -> ("error out"=w378:errorcluster, "Execution UI Out"=w376:refnum<class "Execution UI V2.lvclass">)  [unwired: 8 in]
      }
      event "Test Results": Double Click {
        n156 = event-data() -> ("Tag"=w384:string)  [unwired: 1 in]
        n157 = To Variant(anything=w384) -> (Variant=w383:variant)
        n158 = call "Enqueue Message.vi"("error in (no error)"=w388, "Message Data"=w383, "Message"="Open Front Panel", "Process In"=w389) -> ("error out"=w386:errorcluster, "Process Out"=w387:refnum<class "Execution UI V2.lvclass">)  [unwired: 6 in]
      }
      event "Save": Value Change {
        n159 = event-data() -> ()  [unwired: 1 in, 1 out]
        n160 = call "Enqueue Message.vi"("error in (no error)"=w392, "Message"="Save results", "Process In"=w394) -> ("error out"=w391:errorcluster, "Process Out"=w393:refnum<class "Execution UI V2.lvclass">)  [unwired: 7 in]
      }
      event "Eject": Value Change {
        n161 = event-data() -> ()  [unwired: 1 in, 4 out]
        n162 = call "Enqueue Message.vi"("error in (no error)"=w396, "Message"="Launch Results View", "Process In"=w398) -> ("error out"=w397:errorcluster, "Process Out"=w399:refnum<class "Execution UI V2.lvclass">)  [unwired: 7 in]
      }
      event "Test Results": Value Change {
        n163 = event-data() -> ("NewVal"=w400:string[])  [unwired: 1 in]
        n164 = call "Enqueue Message.vi"("error in (no error)"=w407, "Message Data"=w400, "Message"="Update Description", "Process In"=w408) -> ("error out"=w404:errorcluster, "Process Out"=w403:refnum<class "Execution UI V2.lvclass">)  [unwired: 6 in]
        n165 = call "Enqueue Message.vi"("error in (no error)"=w404, "Message Data"=w400, "Message"="Load Test", "Process In"=w403) -> ("error out"=w406:errorcluster, "Process Out"=w405:refnum<class "Execution UI V2.lvclass">)  [unwired: 6 in]
      }
      event Pane Size {
        # "Set column sizes on pane resize."
        n166 = event-data() -> ()  [unwired: 1 in, 1 out]
        n167 = property on="Test Results" class="Tree (strict)"(error in=w409) -> (error out=w411:errorcluster, "Width"=w412:u32)  [unwired: 1 in, 1 out]
        n168 = Quotient & Remainder(x=w412, y=u32 10) -> (floor(x/y)=w416:u32)  [unwired: 1 out]
        n169 = Multiply(x=w416, y=u32 8) -> (x*y=w413:u32)
        n170 = property on="Test Results" class="Tree (strict)"(error in=w411, "ActiveColNum"=0 ("Active Cell:Active Column Number"), "Width"=w413, "ActiveColNum"=1 ("Active Cell:Active Column Number"), "Width"=w413) -> (error out=w410:errorcluster)  [unwired: 1 in, 1 out]
      }
      event "Test File Path": Value Change {
        # "#TODO"
        # "This case is triggered when running test cases through VI Server.\nTo control test execution from an external VI - get a reference to the \"Test File Path\" control on the User Interface.vi and update the value with the path to test case using a property node."
        n171 = event-data() -> ("NewVal"=w426:path)  [unwired: 1 in]
        n172 = call <vilib>:"Get File Extension.vi"("error in (no error)"=w420, "file"=w426) -> ("error out"=w421:errorcluster, "lowercase file extension"=w422:string, "dup file"=w423:path)  [unwired: 5 in, 2 out]
        n173 = case shown="\"lvclass\"" w422 {
          tunnel: w427 -> [w429 w448 w457]
          tunnel: w421 -> [w428 w447 w456]
          tunnel: w423 -> [_ w442 w454]
          tunnel: [w428 w434 w451] -> w425
          tunnel: [w429 w432 w450] -> w424
          frame Default {
          }
          frame "lvclass" {
            n174 = call "Enqueue Message.vi"("error in (no error)"=w447, "Message Data"=w442, "Message"="Find Tests", "Process In"=w448) -> ("error out"=w438:errorcluster, "Process Out"=w440:refnum<class "Execution UI V2.lvclass">)  [unwired: 6 in]
            n175 = call <vilib>:"Get LV Class Default Value.vi"("error in (no error)"=w438, "class path"=w442) -> ("error out"=w444:errorcluster, "object"=w443:refnum<class>)  [unwired: 8 in]
            n176 = call <vilib>:"Get LV Class Name.vi"("error in (no error)"=w444, "object"=w443) -> ("error out"=w437:errorcluster, "class name"=w431:string)  [unwired: 8 in]
            n177 = Build Array(w431) -> (w436:string[])
            n178 = call "Enqueue Message.vi"("error in (no error)"=w437, "Message Data"=w436, "Message"="Load Test", "Process In"=w440) -> ("error out"=w441:errorcluster, "Process Out"=w439:refnum<class "Execution UI V2.lvclass">)  [unwired: 6 in]
            n179 = call "Enqueue Message.vi"("error in (no error)"=w441, "Message"="Run test suite", "Process In"=w439) -> ("error out"=w435:errorcluster, "Process Out"=w433:refnum<class "Execution UI V2.lvclass">)  [unwired: 7 in]
            n180 = call "Enqueue Message.vi"("error in (no error)"=w435, "Message Data"=w431, "Message"="Set Top Left Tree Node", "Process In"=w433) -> ("error out"=w434:errorcluster, "Process Out"=w432:refnum<class "Execution UI V2.lvclass">)  [unwired: 6 in]
          }
          frame "lvproj" {
            n181 = call "Enqueue Message.vi"("error in (no error)"=w456, "Message Data"=w454, "Message"="Find Tests", "Process In"=w457) -> ("error out"=w452:errorcluster, "Process Out"=w453:refnum<class "Execution UI V2.lvclass">)  [unwired: 6 in]
            n182 = call "Enqueue Message.vi"("error in (no error)"=w452, "Message"="Run all tests", "Process In"=w453) -> ("error out"=w451:errorcluster, "Process Out"=w450:refnum<class "Execution UI V2.lvclass">)  [unwired: 7 in]
          }
        }
      }
      event Menu Selection (User) {
        n183 = event-data() -> ("ItemTag"=w463:string)  [unwired: 1 in]
        n184 = case shown="\"Full size\"" w463 {
          tunnel: w462 -> [w477 w479 w486 w494 w507 w510 w518 w535 w548 w555 w559 w563 w564 w569]
          tunnel: w461 -> [w464 w478 w483 w495 w508 w511 w515 w532 w550 w552 w556 w560 w565 w568]
          tunnel: [w465 w478 w481 w496 w508 w511 w516 w533 w549 w553 w557 w561 w565 w567] -> w460
          tunnel: [w477 w479 w482 w497 w507 w510 w517 w534 w548 w555 w559 w563 w564 w566] -> w459
          frame "Full size" {
            # "This is the same as done in event case for Result Pane: Pane Size, but that case is not trigerd on maximizing window."
            n185 = control-ref of="This VI"() -> (w476:refnum<vi>)
            n186 = property on="Property Node" class="VI"(reference=w476, error in=w464, "FP.State"=T12."Maximized" ("Front Panel Window:State")) -> (error out=w467:errorcluster)  [unwired: 1 out]
            n187 = property on="Test Results" class="Tree (strict)"(error in=w467) -> (error out=w466:errorcluster, "Width"=w474:u32)  [unwired: 1 in, 1 out]
            n188 = Quotient & Remainder(x=w474, y=u32 10) -> (floor(x/y)=w473:u32)  [unwired: 1 out]
            n189 = Multiply(x=w473, y=u32 7) -> (x*y=w472:u32)
            n190 = property on="Test Results" class="Tree (strict)"(error in=w466, "ActiveColNum"=0 ("Active Cell:Active Column Number"), "Width"=w472, "ActiveColNum"=1 ("Active Cell:Active Column Number"), "Width"=w472) -> (error out=w465:errorcluster)  [unwired: 1 in, 1 out]
          }
          frame Default {
          }
          frame "Ignore Inherited Tests" {
            w485 = "Ignore Inherited Tests"
            n191 = Current VI's Menubar() -> (w487:refnum<k9>)
            n192 = Get Menu Item Info(7:w485, 11:w487) -> (4:w484:bool)  [unwired: 1 in, 6 out]
            n193 = Not(x=w484) -> (.not. x?=w480:bool)
            n194 = call "Enqueue Message.vi"("error in (no error)"=w483, "Message Data"=w480, "Message"=w485, "Process In"=w486) -> ("error out"=w481:errorcluster, "Process Out"=w482:refnum<class "Execution UI V2.lvclass">)  [unwired: 6 in]
          }
          frame "Open Project or Test class" {
            n195 = call "File Dialog"("prompt"="Please select a test class or project file to load.", "pattern (all files)"="*.lvclass;*.lvproj;*.lvlib", "pattern label"="Project or class") -> ("selected path"=w493:path, "cancelled"=w489:bool, "error out"=w488:errorcluster)  [unwired: 9 in, 1 out]
            n196 = call <vilib>:"Clear Errors.vi"("error in (no error)"=w488) -> ()  [unwired: 5 in, 2 out]
            n197 = case shown="False" w489 {
              tunnel: [w499 w505] -> w497
              tunnel: [w498 w504] -> w496
              tunnel: w495 -> [w498 w503]
              tunnel: w494 -> [w499 w502]
              tunnel: w493 -> [_ w501]
              frame True {
              }
              frame False {
                n198 = call "Enqueue Message.vi"("error in (no error)"=w503, "Message Data"=w501, "Message"="Find Tests", "Process In"=w502) -> ("error out"=w504:errorcluster, "Process Out"=w505:refnum<class "Execution UI V2.lvclass">)  [unwired: 6 in]
              }
            }
          }
          frame "Configure Test Runner" {
            # "#TODO"
            n199 = One Button Dialog(message="TODO") -> ()  [unwired: 1 in, 1 out]
          }
          frame "Configure Reporting" {
            # "#TODO"
            n200 = One Button Dialog(message="TODO") -> ()  [unwired: 1 in, 1 out]
          }
          frame "Execution Profiler..." {
            n201 = Current VI's Menubar() -> (w513:refnum<k9>)
            n202 = Get Menu Item Info(7:"Execution Profiler...", 11:w513) -> (4:w514:bool)  [unwired: 1 in, 6 out]
            n203 = case shown="False" w514 {
              tunnel: w518 -> [w523 w528]
              tunnel: [w522 w527] -> w517
              tunnel: [w521 w526] -> w516
              tunnel: w515 -> [w520 w525]
              frame False {
                n204 = call "Enqueue Message.vi"("error in (no error)"=w520, "Message"="Enable Execution Profiler", "Process In"=w523) -> ("error out"=w521:errorcluster, "Process Out"=w522:refnum<class "Execution UI V2.lvclass">)  [unwired: 7 in]
              }
              frame True {
                n205 = call "Enqueue Message.vi"("error in (no error)"=w525, "Message"="Disable Execution Profiler", "Process In"=w528) -> ("error out"=w526:errorcluster, "Process Out"=w527:refnum<class "Execution UI V2.lvclass">)  [unwired: 7 in]
              }
            }
          }
          frame "Coverage Analyzer..." {
            n206 = Current VI's Menubar() -> (w530:refnum<k9>)
            n207 = Get Menu Item Info(7:"Coverage Analyzer...", 11:w530) -> (4:w531:bool)  [unwired: 1 in, 6 out]
            n208 = case shown="True" w531 {
              tunnel: w535 -> [w540 w545]
              tunnel: [w539 w544] -> w534
              tunnel: [w538 w543] -> w533
              tunnel: w532 -> [w537 w542]
              frame False {
                n209 = call "Enqueue Message.vi"("error in (no error)"=w537, "Message"="Enable Coverage Analyzer", "Process In"=w540) -> ("error out"=w538:errorcluster, "Process Out"=w539:refnum<class "Execution UI V2.lvclass">)  [unwired: 7 in]
              }
              frame True {
                n210 = call "Enqueue Message.vi"("error in (no error)"=w542, "Message"="Disable Coverage Analyzer", "Process In"=w545) -> ("error out"=w543:errorcluster, "Process Out"=w544:refnum<class "Execution UI V2.lvclass">)  [unwired: 7 in]
              }
            }
          }
          frame "Reset..." {
            n211 = control-ref of="This VI"() -> (w546:refnum<vi>)
            n212 = call "Initialize Controls and Indicators.vi"("error in (no error)"=w550, "VI in"=w546) -> ("error out"=w551:errorcluster)  [unwired: 9 in]
            n213 = control-ref of="This VI"() -> (w547:refnum<vi>)
            n214 = call "Set Front Panel size.vi"("error in (no error)"=w551, "VI in"=w547) -> ("error out"=w549:errorcluster)  [unwired: 9 in]
          }
          frame "Documentation..." {
            n215 = call-poly <vilib>:"Open URL in Default Browser.vi"("error in (no error)"=w552, "URL"="https://astemes.github.io/astemes-lunit/") -> ("error out"=w553:errorcluster)  [unwired: 4 in, 1 out]
          }
          frame "Report issue..." {
            n216 = call-poly <vilib>:"Open URL in Default Browser.vi"("error in (no error)"=w556, "URL"="https://github.com/astemes/astemes-lunit/issues") -> ("error out"=w557:errorcluster)  [unwired: 4 in, 1 out]
          }
          frame "Post an Idea..." {
            n217 = call-poly <vilib>:"Open URL in Default Browser.vi"("error in (no error)"=w560, "URL"="https://www.vipm.io/post/suggestion/?package_name=astemes_lib_lunit&return_url=/package/astemes_lib_lunit/") -> ("error out"=w561:errorcluster)  [unwired: 4 in, 1 out]
          }
          frame "About" {
            n218 = call "About Dialog.vi"() -> ()  [unwired: 12 in]
          }
          frame "Exit" {
            n219 = call-dynamic "Stop.vi"("error in (no error)"=w568, "Execution UI In"=w569) -> ("error out"=w567:errorcluster, "Execution UI Out"=w566:refnum<class "Execution UI V2.lvclass">)  [unwired: 7 in, 1 out]
          }
        }
      }
      event User Event {
        n220 = event-data() -> ()  [unwired: 1 in, 4 out]
      }
      event Panel Close? {
        w577 = TRUE  # Discard?
        n221 = event-data() -> ()  [unwired: 1 in, 4 out]
        n222 = call-dynamic "Stop.vi"("error in (no error)"=w573, "Execution UI In"=w576) -> ("error out"=w574:errorcluster, "Execution UI Out"=w575:refnum<class "Execution UI V2.lvclass">)  [unwired: 7 in, 1 out]
        n223 = event-data ("Event Filter Node")("Discard?"=w577) -> ()  [unwired: 1 in, 1 out]
      }
    }
    n224 = call "Handle Process Errors.vi"("error in (no error)"=w304, "Process In"=w309) -> ("error out"=w303:errorcluster, "Process Out"=w305:refnum<class "Execution UI V2.lvclass">)  [unwired: 8 in]
  }
  n225 = Unregister For Events(event registration refnum=w9, error in=w4) -> (error out=w2:errorcluster)
  n226 = Merge Errors(w2, w7) -> (→"error out":errorcluster)
